vi "example_vi_3.vi"() -> ()   [LabVIEW 2015]
panel:
  out "new number":dbl
  in  "starting number":dbl
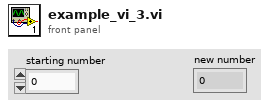
[diagram p1: front panel]
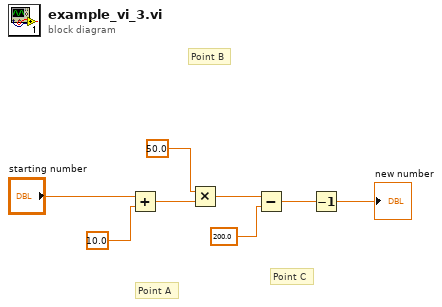
[diagram p0: block diagram]
diagram:
  # "Point C"
  # "Point B"
  # "Point A"
  n1 = Add(x="starting number", y=10.0) -> (x+y=w6:dbl)
  n2 = Multiply(x=50.0, y=w6) -> (x*y=w5:dbl)
  n3 = Subtract(x=w5, y=200.0) -> (x-y=w4:dbl)
  n4 = Decrement(x=w4) -> (x-1=→"new number":dbl)
